vi "niRFUtil FTW Generate RRC FIR Filter.vi"(1 "Alpha":T1=0.01 format="%.3g", 2 "Minimum Selectivity (dB)":dbl=70.0 format="%.2f", 3 "Sampling Rate (Hz)":dbl=1.0 format="%^.3e", 4 "Bandwidth (Hz)":dbl=1.0 format="%^.3e") -> (0 "Filter":T2={"x0"=0.0, "dx"=1.0, "y"=[]} {"y" min=0 max=127 format="%.2f"; "dx" format="%^.2e"; "x0" format="%^.2e"})   [LabVIEW 2015, in "niRFUtil.lvlib"]
doc: "(c) Copyright 2006, National Instruments, Inc. This VI may not be duplicated, sold, or distributed without written consent from National Instruments."
uses:
  niRFUtil.lvlib
  Includes/niRFUtil INC Real Waveform.ctl
  Includes/niRFUtil INC Real Array.ctl
  Includes/niRFUtil INC RRC Filter Alpha.ctl
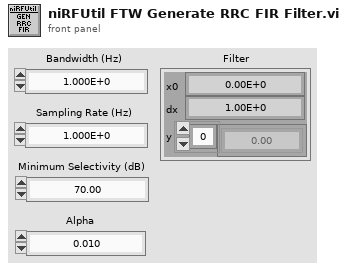
[diagram p1: front panel]
types:
  T1 = typedef "niRFUtil.lvlib/niRFUtil INC RRC Filter Alpha.ctl" = dbl
  T2 = typedef "niRFUtil.lvlib/niRFUtil INC Real Waveform.ctl" = cluster{"x0":dbl, "dx":dbl, "y":T3}
  T3 = typedef "niRFUtil.lvlib/niRFUtil INC Real Array.ctl" = sgl[]
  T4 = cluster{"Alpha":T1, "Minimum Selectivity (dB)":dbl, "Bandwidth (Hz)":dbl, "Sampling Rate (Hz)":dbl}
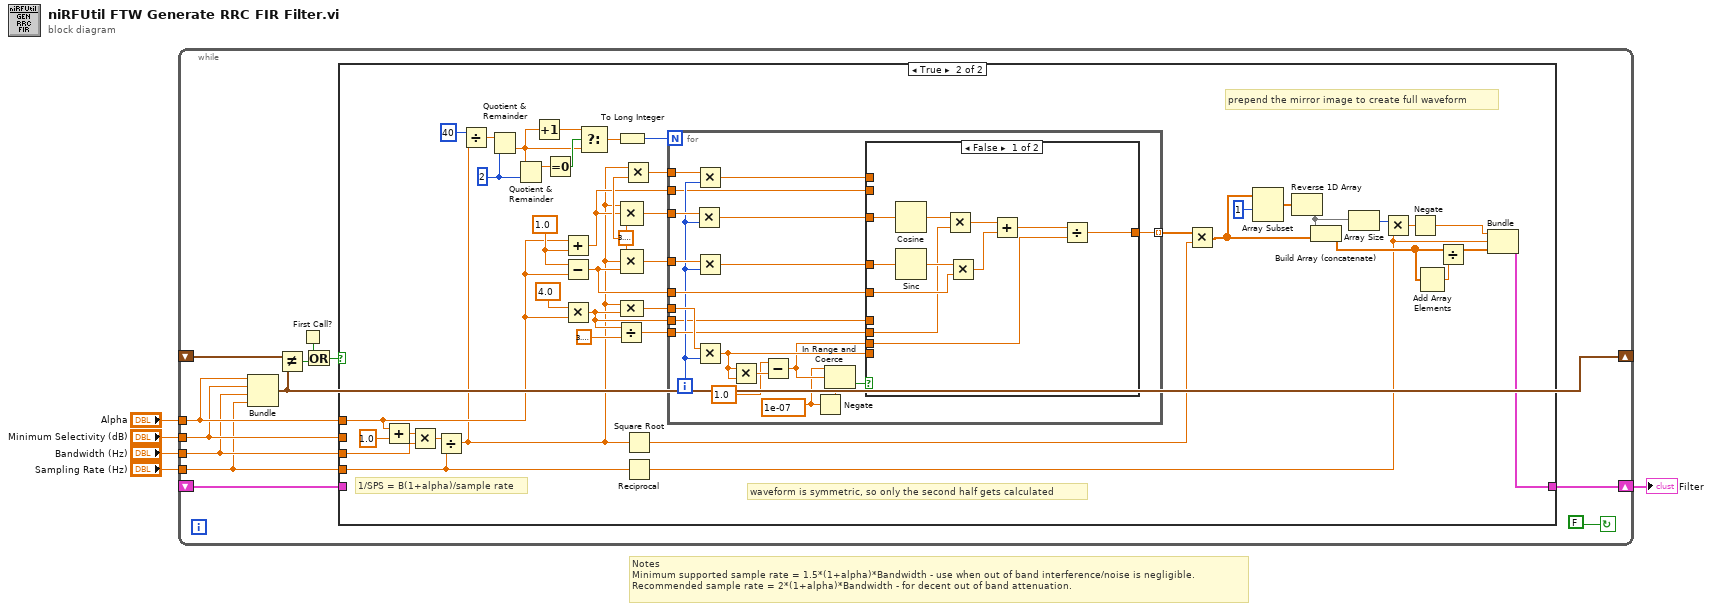
[diagram p0: block diagram]
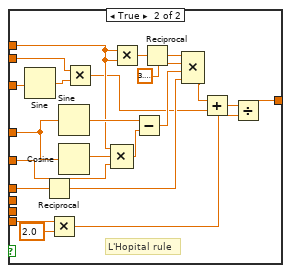
[diagram p3: hidden frame]
diagram:
  # "Notes\nMinimum supported sample rate = 1.5*(1+alpha)*Bandwidth - use when out of band interference/noise is negligible.\nRecommended sample rate = 2*(1+alpha)*Bandwidth - for decent out of band attenuation."
  n1 = while {
    shift-right: [w13] -> _
    shift-left: _ -> [w14]
    tunnel: "Alpha" -> [w9]
    shift-right: [w10] -> w5
    shift-left: _ -> [w15]
    tunnel: "Sampling Rate (Hz)" -> [w6]
    tunnel: "Minimum Selectivity (dB)" -> [w8]
    tunnel: "Bandwidth (Hz)" -> [w7]
    stop <- FALSE ("reset? (T)") continue-if-true
    n2 = Bundle("Alpha"=w9, "Minimum Selectivity (dB)"=w8, "Bandwidth (Hz)"=w7, "Sampling Rate (Hz)"=w6) -> (w13:T4)  [unwired: 1 out]
    n3 = Not Equal?(x=w14, y=w13) -> (x != y?=w12:bool)
    n4 = First Call?() -> (First Call?: T/F=w16:bool)
    n5 = Or(x=w16, y=w12) -> (x .or. y?=w11:bool)
    n6 = case shown="True" w11 {
      tunnel: w9 -> [_ w34]
      tunnel: [w18 w57] -> w10
      tunnel: w15 -> [w18 _]
      tunnel: w6 -> [_ w29]
      tunnel: w8 -> [_ _]
      tunnel: w7 -> [_ w31]
      frame False {
      }
      frame True {
        w53 = 3.141592653589793
        w54 = 1.0 ("y")
        w24 = 2 ("y")
        # "1/SPS = B(1+alpha)/sample rate"
        # "waveform is symmetric, so only the second half gets calculated"
        # "prepend the mirror image to create full waveform"
        n7 = Add(x=w34, y=T1 1.0) -> (x+y=w32:T1)
        n8 = Multiply(x=w32, y=w31) -> (x*y=w30:T1)
        n9 = Divide(x=w30, y=w29) -> (x/y=w27:T1)
        n10 = Divide(x=40 ("y"), y=w27) -> (x/y=w26:T1)
        n11 = Quotient & Remainder(x=w26, y=w24) -> (floor(x/y)=w21:T1)  [unwired: 1 out]
        n12 = Quotient & Remainder(x=w21, y=w24) -> (x-y*floor(x/y)=w23:T1)  [unwired: 1 out]
        n13 = Increment(x=w21) -> (x+1=w20:T1)
        n14 = Equal To 0?(x=w23) -> (x = 0?=w22:bool)
        n15 = Add(x=w34, y=w54) -> (x+y=w38:T1)
        n16 = Subtract(x=w54, y=w34) -> (x-y=w48:T1)
        n17 = Multiply(x=4.0 ("Input"), y=w34) -> (x*y=w39:T1)
        n18 = Select(t=w20, s=w22, f=w21) -> (s? t:f=w19:T1)
        n19 = Divide(x=w39, y=3.141592653589793) -> (x/y=w46:T1)
        n20 = To Long Integer(number=w19) -> (32bit integer=w25:i32)
        n21 = Compound Arithmetic op=MULTIPLY(w27, w38, w53) -> (w52:T1)
        n22 = Compound Arithmetic op=MULTIPLY(w53, w27, w48) -> (w51:T1)
        n23 = Compound Arithmetic op=MULTIPLY(w27, w39) -> (w50:T1)
        n24 = Multiply(x=w27, y=w53) -> (x*y=w40:T1)
        n25 = Square Root(x=w27) -> (sqrt(x)=w44:T1)
        n26 = Reciprocal(x=w29) -> (1/x=w35:dbl)
        n27 = for {
          N: w25 -> [_]
          tunnel: w52 -> [w78]
          tunnel: w51 -> [w79]
          tunnel: w50 -> [w80]
          tunnel: w48 -> [w73]
          tunnel: w46 -> [w72]
          tunnel: [w71] -> w45 mode=indexing
          tunnel: w40 -> [w70]
          tunnel: w39 -> [w67]
          tunnel: w38 -> [w66]
          i -> [w69]
          w62 = 1e-07 ("y")
          n28 = Multiply(x=w78, y=w69) -> (x*y=w77:T1)
          n29 = Multiply(x=w70, y=w69) -> (x*y=w68:T1)
          n30 = Multiply(x=w79, y=w69) -> (x*y=w76:T1)
          n31 = Multiply(x=w80, y=w69) -> (x*y=w65:T1)
          n32 = Multiply(x=w65, y=w65) -> (x*y=w75:T1)
          n33 = Subtract(x=1.0 ("y"), y=w75) -> (x-y=w63:T1)
          n34 = Negate(x=w62) -> (-x=w61:dbl)
          n35 = In Range and Coerce(upper limit=w62, x=w63, lower limit=w61) -> (In Range?=w64:bool)  [unwired: 1 out]
          n36 = case shown="False" w64 {
            tunnel: w77 -> [w91 w102]
            tunnel: w76 -> [w90 w113]
            tunnel: w73 -> [w88 w92]
            tunnel: w72 -> [w86 _]
            tunnel: w63 -> [w82 _]
            tunnel: [w81 w93] -> w71
            tunnel: w68 -> [_ w109]
            tunnel: w67 -> [_ w105]
            tunnel: w66 -> [_ w100]
            tunnel: w65 -> [_ w96]
            frame False {
              n37 = Cosine(x=w91) -> (cos(x)=w87:T1)
              n38 = Sinc(1:w90) -> (0:w89:T1)
              n39 = Multiply(x=w87, y=w86) -> (x*y=w85:T1)
              n40 = Multiply(x=w89, y=w88) -> (x*y=w84:T1)
              n41 = Add(x=w85, y=w84) -> (x+y=w83:T1)
              n42 = Divide(x=w83, y=w82) -> (x/y=w81:T1)
            }
            frame True {
              # "L'Hopital rule"
              n43 = Sine(x=w102) -> (sin(x)=w101:T1)
              n44 = Reciprocal(x=w105) -> (1/x=w104:T1)
              n45 = Multiply(x=w96, y=2.0) -> (x*y=w94:T1)
              n46 = Sine(x=w113) -> (sin(x)=w112:T1)
              n47 = Cosine(x=w113) -> (cos(x)=w110:T1)
              n48 = Multiply(x=w100, y=w101) -> (x*y=w98:T1)
              n49 = Compound Arithmetic op=MULTIPLY(w109, w110, w92) -> (w111:T1)
              n50 = Multiply(x=w109, y=w109) -> (x*y=w108:T1)
              n51 = Subtract(x=w112, y=w111) -> (x-y=w103:T1)
              n52 = Reciprocal(x=w108) -> (1/x=w107:T1)
              n53 = Compound Arithmetic op=MULTIPLY(w107, 3.141592653589793, w103, w104) -> (w99:T1)
              n54 = Add(x=w99, y=w98) -> (x+y=w97:T1)
              n55 = Divide(x=w97, y=w94) -> (x/y=w93:T1)
            }
          }
        }
        n56 = Multiply(x=w45, y=w44) -> (x*y=w41:T1[])
        n57 = Array Subset(array=w41, index=1 ("Array Index")) -> (w42:T1[])  [unwired: 1 in]
        n58 = Reverse 1D Array(array=w42) -> (reversed array=w37:T1[])
        n59 = Build Array (concatenate)(w37, w41) -> (w36:T1[])
        n60 = Array Size(array=w37) -> (size(s)=w60:i32)
        n61 = Multiply(x=w60, y=w35) -> (x*y=w59:dbl)
        n62 = Negate(x=w59) -> (-x=w58:dbl)
        n63 = Add Array Elements(numeric array=w36) -> (sum=w56:T1)
        n64 = Divide(x=w36, y=w56) -> (x/y=w55:T1[])
        n65 = Bundle(w58, w35, w55) -> (w57:cluster{dbl, dbl, T1[]})  [unwired: 1 in]
      }
    }
  }
  "Filter" <- w5
